vi "Acquire Humidity.vi"(8 "error in (no error)":errorcluster, 11 "ARS-0220 in":refnum<class "ARS-0220.lvclass">) -> (0 "error out":errorcluster, 2 "Humidity Data":T1, 3 "ARS-0220 out":refnum<class "ARS-0220.lvclass">)   [LabVIEW 2021, in "Environment Chamber.lvlib" / "ARS-0220.lvclass"]
uses:
  ARS-0220.lvclass
  ARS-0220.lvclass/ARS-0220.ctl
  Support Libraries/Climatic Chamber/Climatic Chamber.lvlib
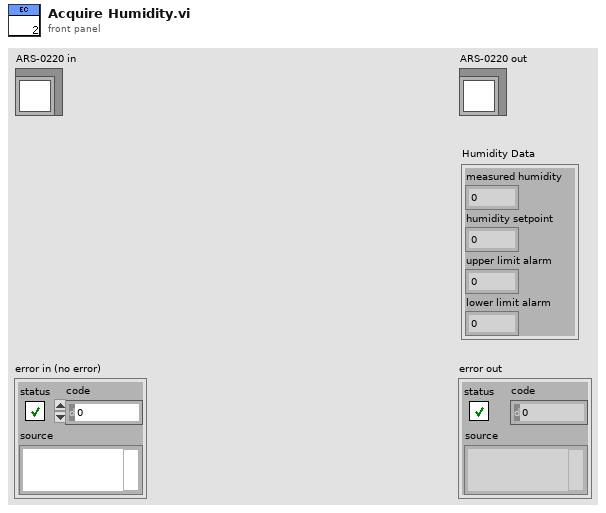
[diagram p1: front panel]
types:
  T1 = cluster{"measured humidity":dbl, "humidity setpoint":dbl, "upper limit alarm":dbl, "lower limit alarm":dbl}
  T2 = cluster{"measured temp":dbl, "temp setpoint":dbl, "upper limit alarm":dbl, "lower limit alarm":dbl}
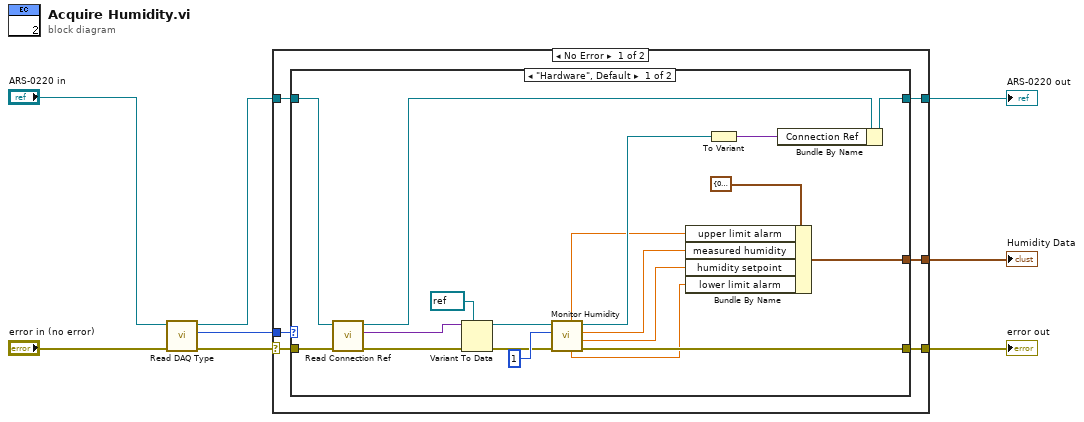
[diagram p0: block diagram]
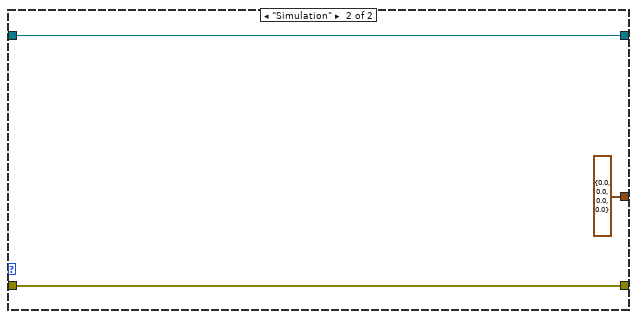
[diagram p2: hidden frame]
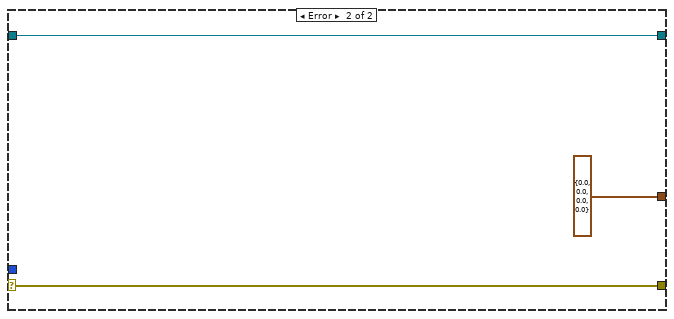
[diagram p3: hidden frame]
diagram:
  n1 = call "Read DAQ Type.vi"("error in (no error)"="error in (no error)", "ARS-0220 in"="ARS-0220 in") -> ("error out"=w8:errorcluster, "DAQ Type"=w7:enum16{"Hardware", "Simulation"}, "ARS-0220 out"=w1:refnum<class "ARS-0220.lvclass">)  [unwired: 7 in]
  n2 = case shown="No Error" w8 {
    selector: w8 -> [w13 w38]
    tunnel: w1 -> [w12 w39]
    tunnel: w7 -> [w14 _]
    tunnel: [w11 w39] -> w5
    tunnel: [w10 w38] -> w4
    tunnel: [w9 T2 {"measured temp"=0.0, "temp setpoint"=0.0, "upper limit alarm"=0.0, "lower limit alarm"=0.0} ("Temp Data")] -> w2
    frame No Error {
      n3 = case shown="\"Hardware\", Default" w14 {
        tunnel: w13 -> [w32 w35]
        tunnel: w12 -> [w17 w36]
        tunnel: [w26 w36] -> w11
        tunnel: [w24 w35] -> w10
        tunnel: [w18 T1 {"measured humidity"=0.0, "humidity setpoint"=0.0, "upper limit alarm"=0.0, "lower limit alarm"=0.0} ("Humidity Data")] -> w9
        frame "Hardware", Default {
          n4 = call "Read Connection Ref.vi"("error in (no error)"=w32, "ARS-0220 in"=w17) -> ("error out"=w31:errorcluster, "Connection Ref"=w29:variant, "ARS-0220 out"=w16:refnum<class "ARS-0220.lvclass">)  [unwired: 7 in]
          n5 = Variant To Data(error in=w31, type=refnum<visa-resource-name> refnum ("VISA resource name"), Variant=w29) -> (data=w27:refnum<visa-resource-name>, error out=w30:errorcluster)
          n6 = call "Monitor Humidity.vi"("error in (no error)"=w30, "Address (0)"=1, "VISA resource name"=w27) -> ("error out"=w24:errorcluster, "humidity setpoint"=w21:dbl, "measured humidity"=w22:dbl, "VISA resource name out"=w25:refnum<visa-resource-name>, "lower limit alarm"=w20:dbl, "upper limit alarm"=w23:dbl)  [unwired: 3 in]
          n7 = Bundle By Name(cluster=T1 {"measured humidity"=0.0, "humidity setpoint"=0.0, "upper limit alarm"=0.0, "lower limit alarm"=0.0} ("Humidity Data"), "upper limit alarm"=w23, "measured humidity"=w22, "humidity setpoint"=w21, "lower limit alarm"=w20) -> (w18:T1)
          n8 = To Variant(anything=w25) -> (Variant=w15:variant)
          n9 = Bundle By Name(cluster=w16, "Connection Ref"=w15) -> (w26:refnum<class "ARS-0220.lvclass">)
        }
        frame "Simulation" {
        }
      }
    }
    frame Error {
    }
  }
  "error out" <- w4
  "ARS-0220 out" <- w5
  "Humidity Data" <- w2
